vi "setup file.vi"(4 "sampling rate":dbl, 5 "accel range":dbl, 6 "counts per rev":dbl, 7 "gyro range":dbl, 8 "error in (no error)":errorcluster, 11 "selected path":path) -> (0 "error out":errorcluster, 1 "channel names":string[](array[string]), 3 "tdms file out":refnum<k34>)   [LabVIEW 2013]
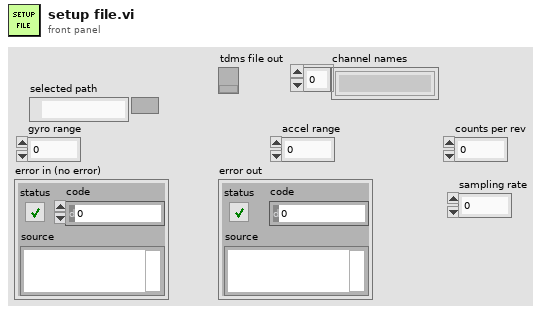
[diagram p1: front panel]
types:
  T1 = enum16{"open", "open or create", "create or replace", "create", "open (read-only)"}
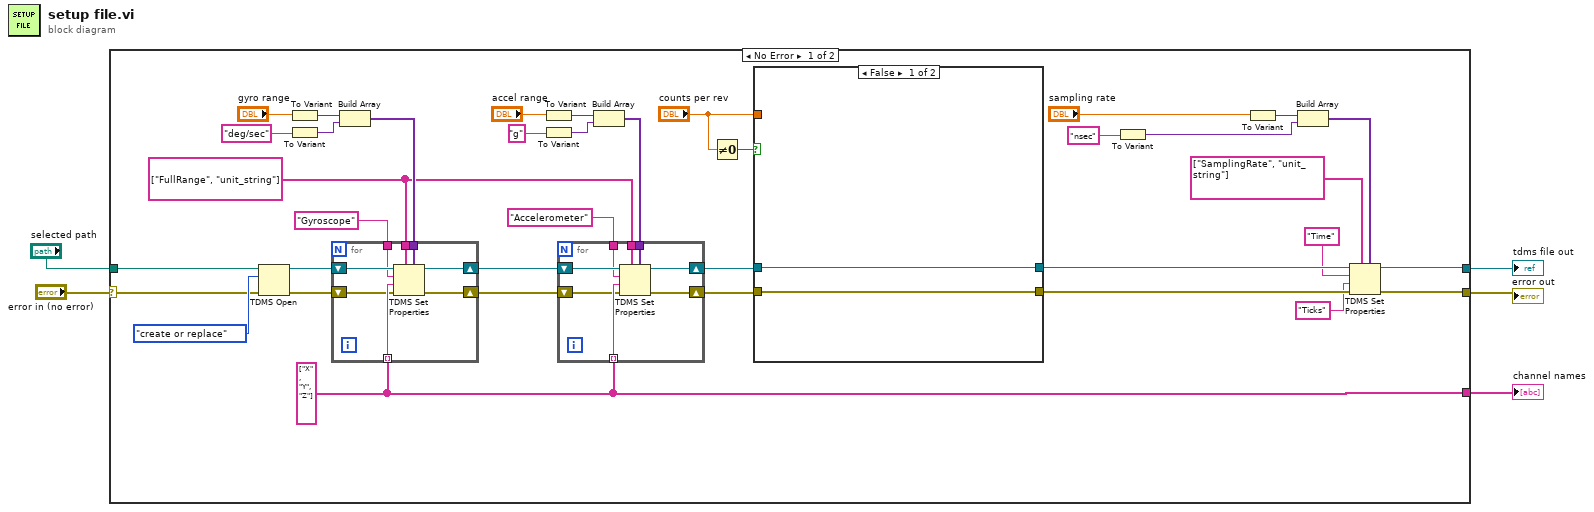
[diagram p0: block diagram]
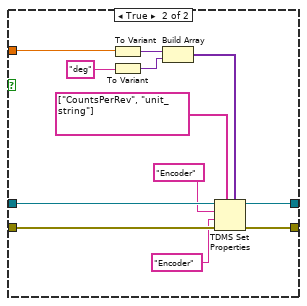
[diagram p2: hidden frame]
diagram:
  n1 = case shown="No Error" "error in (no error)" {
    selector: "error in (no error)" -> [w23 w73]
    tunnel: "selected path" -> [w41 _]
    tunnel: [w14 _] -> w3
    tunnel: [w13 w73] -> w2
    tunnel: [w22 _] -> w1
    frame No Error {
      w29 = string[] ["FullRange", "unit_string"] ("property names")
      w22 = string[] ["X", "Y", "Z"] ("channel name(s)")
      n2 = TDMS Open(8:w23, 10:T1."create or replace" ("operation (0:open)"), 11:w41) -> (0:w38:errorcluster, 3:w40:refnum<k34>)  [unwired: 4 in]
      n3 = To Variant(anything="gyro range") -> (Variant=w35:variant)
      n4 = To Variant(anything="deg/sec" ("group name (Untitled)")) -> (Variant=w34:variant)
      n5 = Build Array(w35, w34) -> (w33:variant[])
      n6 = for {
        tunnel: "Gyroscope" ("group name (Untitled)") -> [w71]
        tunnel: w22 -> [w70] mode=indexing
        shift-right: [w68] -> w30
        shift-left: w38 -> [w69]
        tunnel: w29 -> [w67]
        tunnel: w33 -> [w66]
        shift-right: [w65] -> w31
        shift-left: w40 -> [w72]
        n7 = TDMS Set Properties(5:w66, 7:w67, 8:w69, 9:w70, 10:w71, 11:w72) -> (0:w68:errorcluster, 3:w65:refnum<k34>)  [unwired: 2 out]
      }
      n8 = To Variant(anything="accel range") -> (Variant=w27:variant)
      n9 = To Variant(anything="g" ("group name (Untitled)")) -> (Variant=w28:variant)
      n10 = Build Array(w27, w28) -> (w24:variant[])
      n11 = for {
        tunnel: "Accelerometer" ("group name (Untitled)") -> [w63]
        tunnel: w22 -> [w62] mode=indexing
        shift-right: [w60] -> w20
        shift-left: w30 -> [w61]
        tunnel: w29 -> [w59]
        tunnel: w24 -> [w58]
        shift-right: [w57] -> w21
        shift-left: w31 -> [w64]
        n12 = TDMS Set Properties(5:w58, 7:w59, 8:w61, 9:w62, 10:w63, 11:w64) -> (0:w60:errorcluster, 3:w57:refnum<k34>)  [unwired: 2 out]
      }
      n13 = Not Equal To 0?(x="counts per rev") -> (x != 0?=w18:bool)
      n14 = case shown="False" w18 {
        tunnel: w21 -> [w44 w56]
        tunnel: [w44 w55] -> w16
        tunnel: w20 -> [w43 w54]
        tunnel: [w43 w53] -> w15
        tunnel: "counts per rev" -> [_ w52]
        frame False {
        }
        frame True {
          n15 = To Variant(anything=w52) -> (Variant=w50:variant)
          n16 = To Variant(anything="deg" ("group name (Untitled)")) -> (Variant=w49:variant)
          n17 = Build Array(w50, w49) -> (w48:variant[])
          n18 = TDMS Set Properties(5:w48, 7:string[] ["CountsPerRev", "unit_string"] ("property names"), 8:w54, 9:"Encoder" ("group name"), 10:"Encoder" ("group name"), 11:w56) -> (0:w53:errorcluster, 3:w55:refnum<k34>)  [unwired: 2 out]
        }
      }
      n19 = To Variant(anything="nsec" ("group name (Untitled)")) -> (Variant=w6:variant)
      n20 = To Variant(anything="sampling rate") -> (Variant=w12:variant)
      n21 = Build Array(w12, w6) -> (w11:variant[])
      n22 = TDMS Set Properties(5:w11, 7:string[] ["SamplingRate", "unit_string"] ("property names"), 8:w15, 9:"Ticks" ("group name"), 10:"Time" ("group name"), 11:w16) -> (0:w13:errorcluster, 3:w14:refnum<k34>)  [unwired: 2 out]
    }
    frame Error {
    }
  }
  "tdms file out" <- w3
  "error out" <- w2
  "channel names" <- w1
